vi "Add To Profile.vi"(10 "Profile":string, 11 "Descriptor":string) -> (3 "Flavoured Descriptor":string)   [LabVIEW 2015]
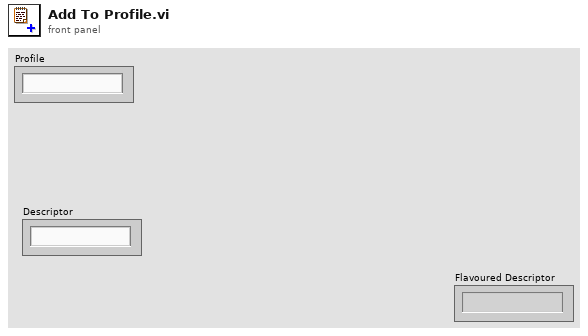
[diagram p1: front panel]
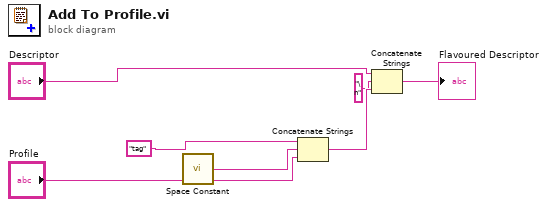
[diagram p0: block diagram]
diagram:
  n1 = call <vilib>:"Space Constant.vi"() -> ("String"=w2:string)
  n2 = Concatenate Strings("tag", w2, "Profile") -> (w4:string)
  n3 = Concatenate Strings("Descriptor", "\n" ("string"), w4) -> (→"Flavoured Descriptor":string)
